vi "禹山叶绿素a校准.vi"() -> ()   [LabVIEW 2016, in "斯坦道多参数.lvlib"]
uses:
  <vilib>/Utility/miscctls.llb/LVPointTypeDef.ctl
  <vilib>/Analysis/NI_AALBase.lvlib
  <vilib>/Analysis/NI_AALPro.lvlib
  <vilib>/Utility/config.llb/NI_LVConfig.lvlib
panel:
  out "通讯状态":string
  out "第二点校准值":dbl
  out "第一点校准值":dbl
  out "最小值":sgl format="%.2g"
  out "最大值":sgl format="%.2g"
  in  "校准停止":bool
  in  "校准模式":enum16{"两点校准", "单点校准"}(ring)
  in  "标液2":dbl
  in  "标液1":dbl
  out "波形图表":sgl(graph) caption="历史曲线"
  out "温度测量值":dbl caption="温度" format="%#.2f"
  out "变异系数":dbl format="%.6g"
  out "standard deviation":dbl caption="标准差" format="%0.2f"
  out "mean":dbl caption="均值" format="%0.2f"
  out "提示":string
  in  "校准启动":bool
  out "测试值":dbl format="%#.2f"
  out "电极斜率":dbl format="%#.6f"
  out "电极零点":dbl format="%#.6f"
  # "叶绿素a电极设定"
  # "请选择校准模式:"
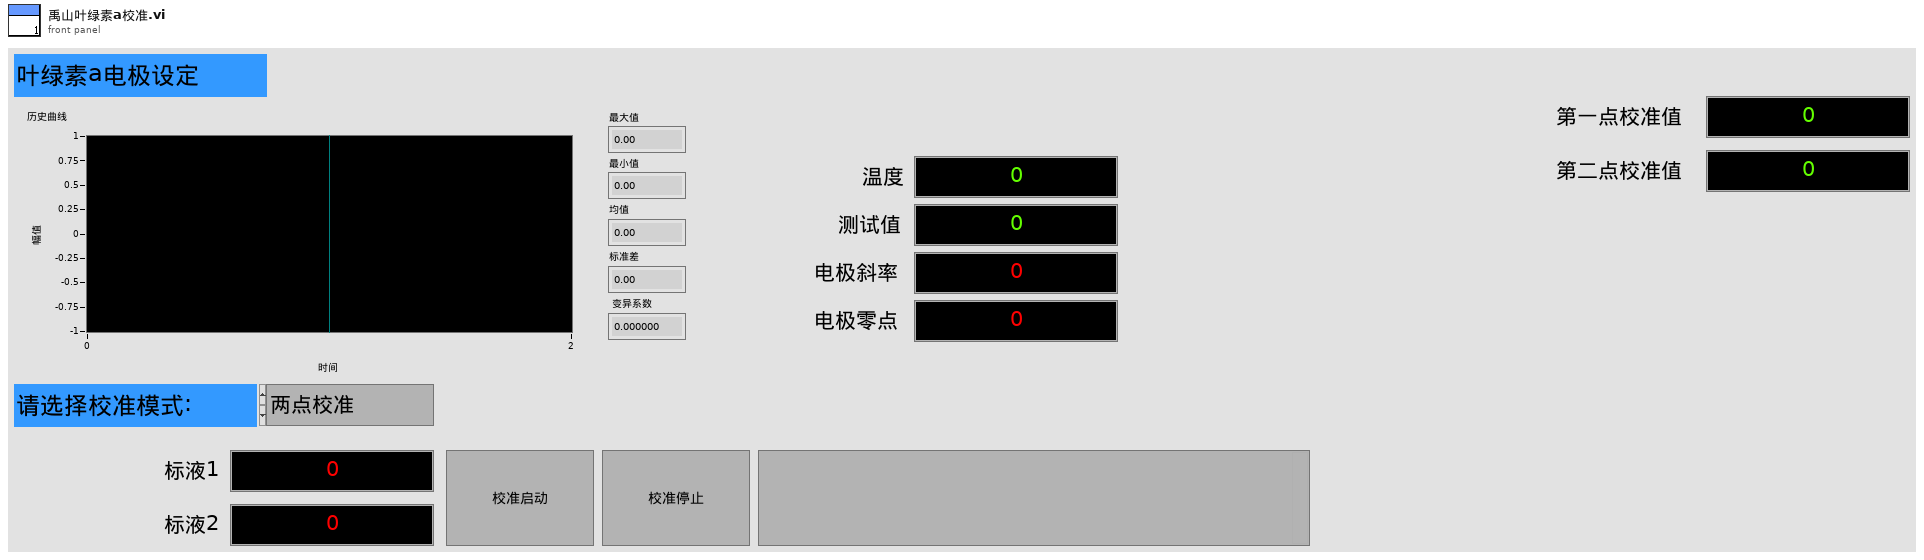
[diagram p1: front panel]
types:
  T1 = typedef "斯坦道多参数.lvlib/校准步骤.ctl" = enum16{"待机", "放置第一点标液", "第一点校准启动", "第一点校准写入", "第一点校准失败", "放置第二点标液", "第二点校准启动", "第二点校准写入", "第二点校准失败", "放置第三点标液", "第三点校准启动", "第三点校准写入", "第三点校准失败", "校准结果写入", "校准结束"}
  T2 = typedef "LVPointTypeDef.ctl" = cluster{"Horizontal":i16, "Vertical":i16}
  T3 = typedef "NI_LVConfig.lvlib/Config Data RefNum.ctl" = refnum<k1>
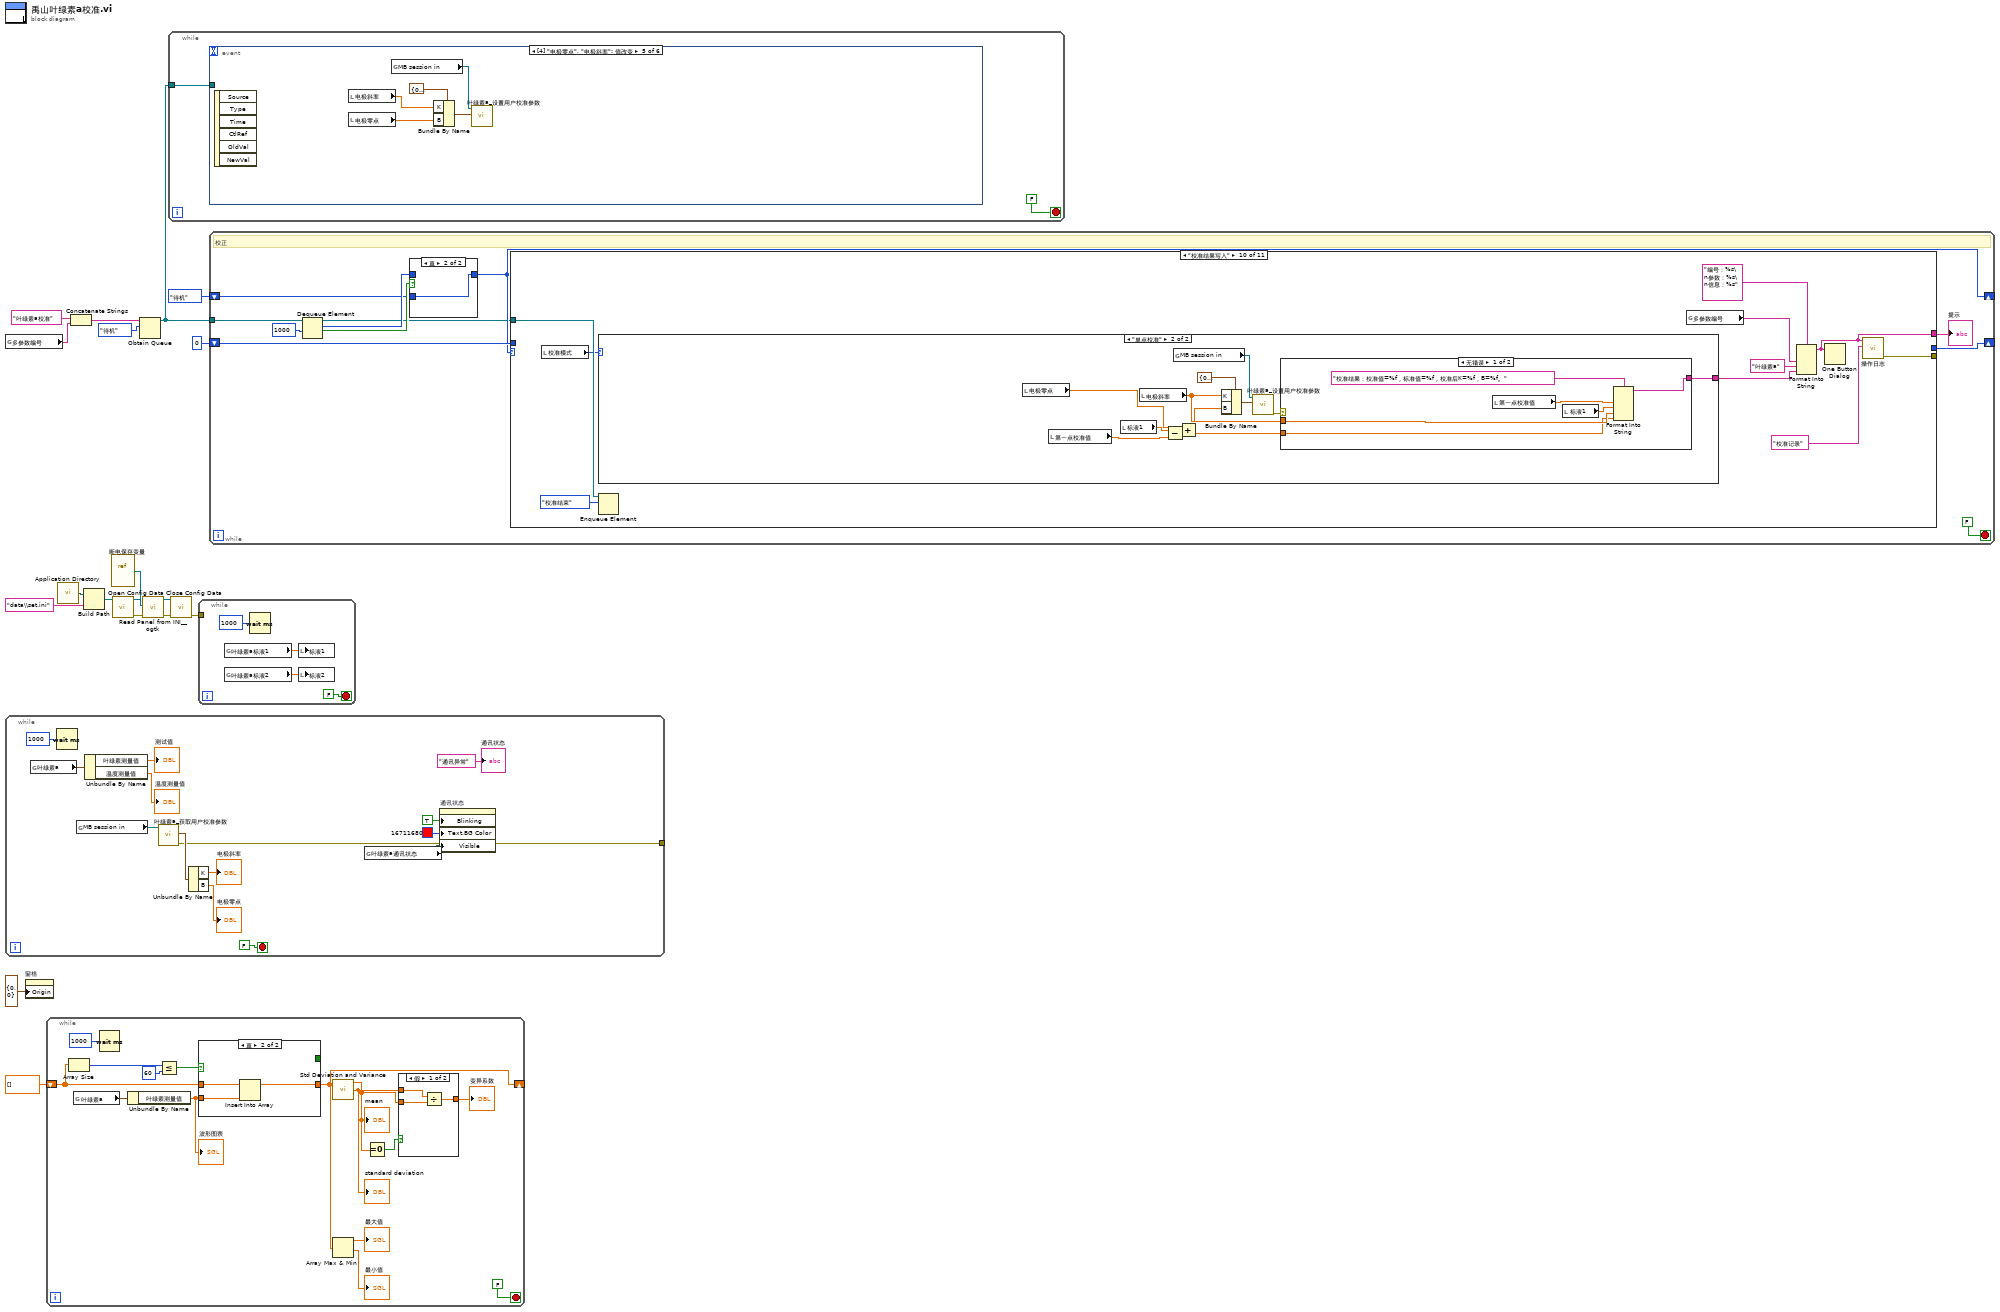
[diagram p0: block diagram]
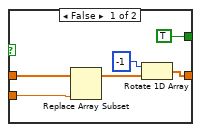
[diagram p3: hidden frame]
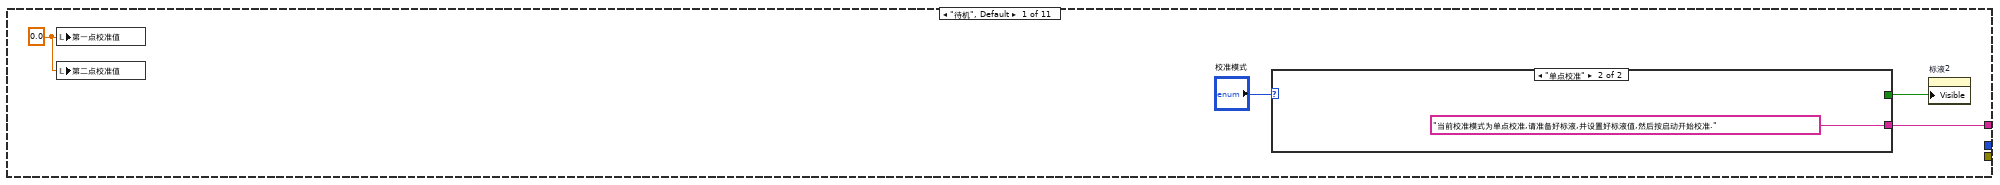
[diagram p5: hidden frame]
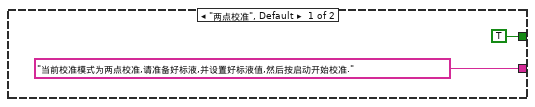
[diagram p6: hidden frame]
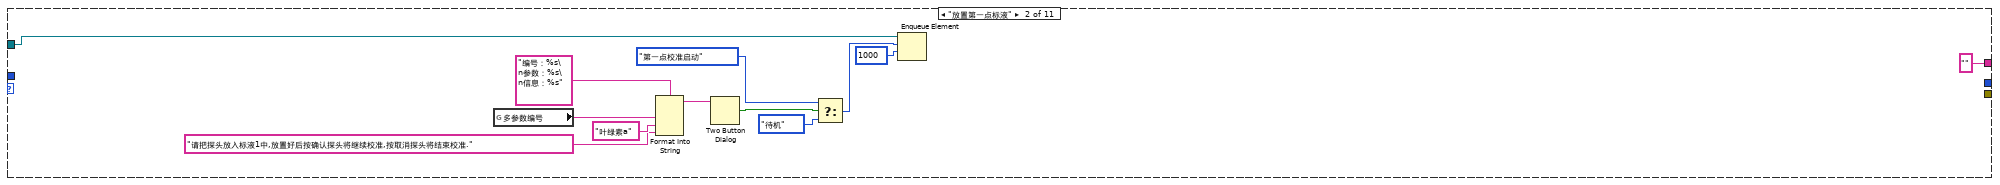
[diagram p7: hidden frame]
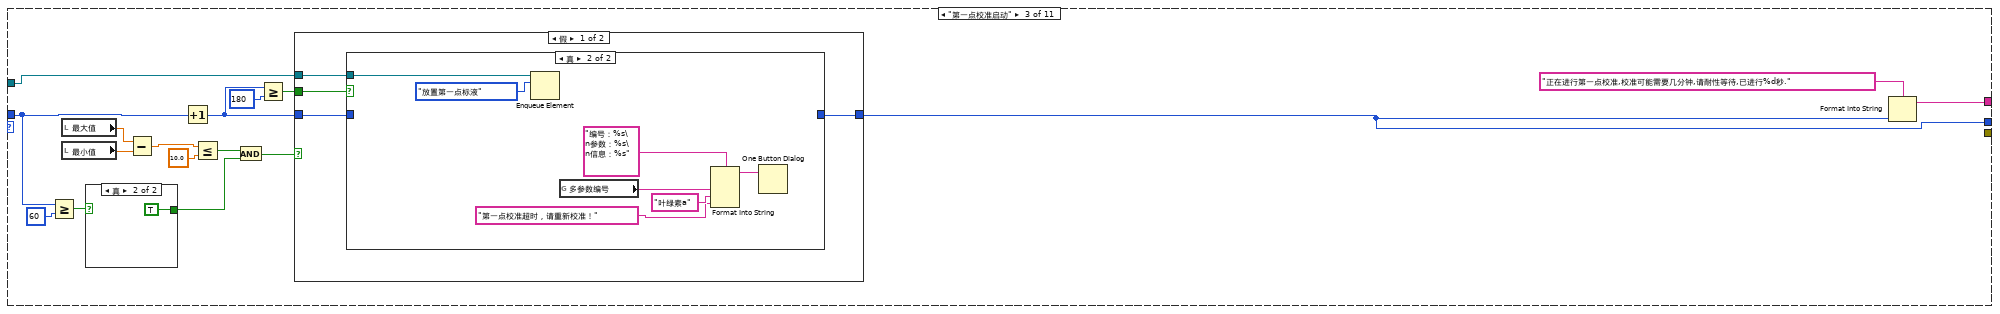
[diagram p8: hidden frame]
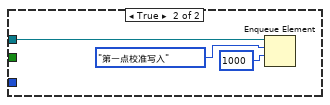
[diagram p10: hidden frame]
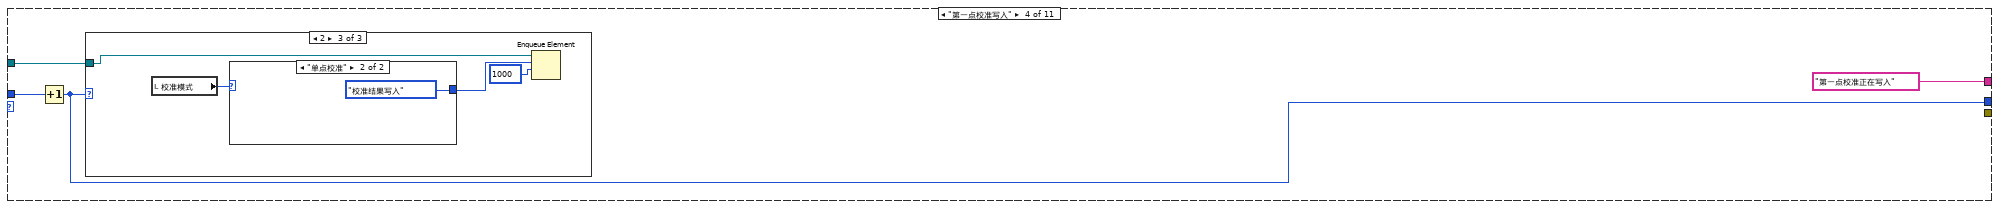
[diagram p12: hidden frame]
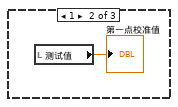
[diagram p14: hidden frame]
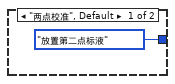
[diagram p15: hidden frame]
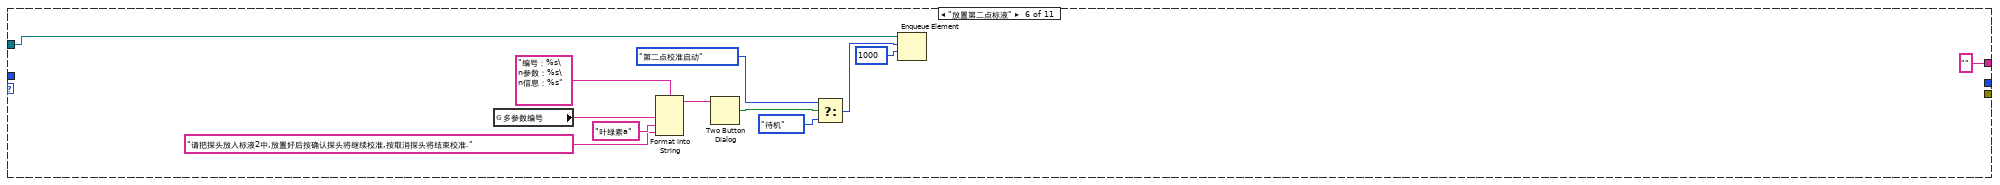
[diagram p17: hidden frame]
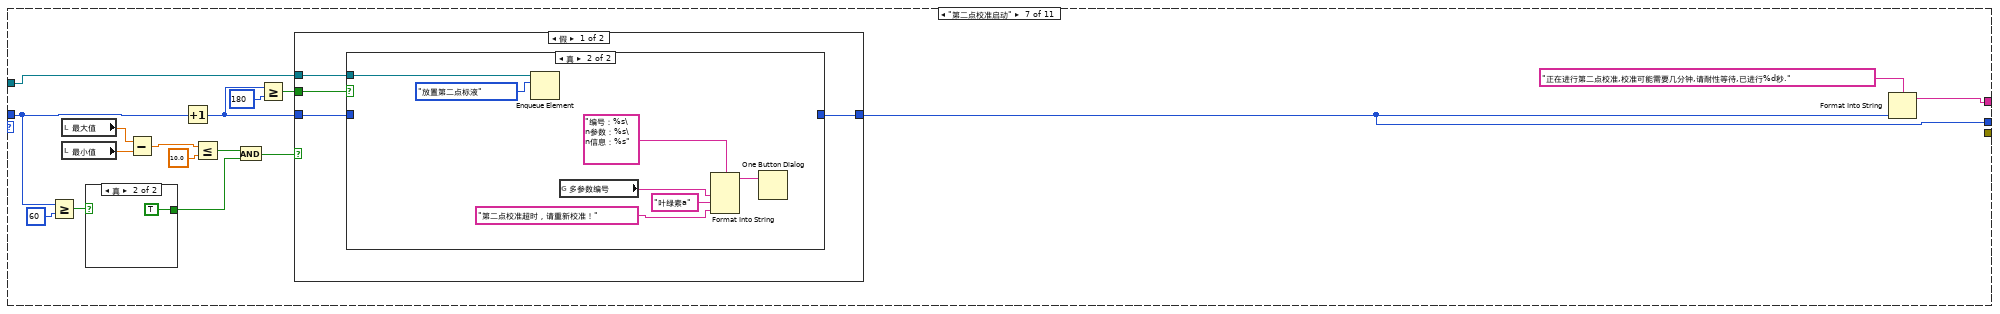
[diagram p18: hidden frame]
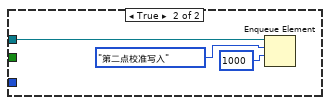
[diagram p20: hidden frame]
diagram:
  n1 = global read "多参数全局变量.vi" "多参数编号"() -> (w1:string)
  n2 = while {
    tunnel: [w27] -> _
    stop <- FALSE stop-if-true
    n3 = global read "禹山过程全局变量.vi" "叶绿素a"() -> (w24:cluster{"温度测量值":sgl, "叶绿素测量值":sgl, "错误标志":u16})
    n4 = Wait (ms)(milliseconds to wait=u32 1000 ("等待时间（毫秒）")) -> ()  [unwired: 1 out]
    n5 = global read "多参数全局变量.vi" "MB session in"() -> (w23:refnum<class "MB_Master.lvclass">)
    n6 = Unbundle By Name(w24) -> ("叶绿素测量值"=→"测试值":sgl, "温度测量值"=→"温度测量值":sgl)
    n7 = call "叶绿素a_获取用户校准参数.vi"("MB session in"=w23) -> ("error out"=w27:errorcluster, "输出值"=w30:cluster{"K":sgl, "B":sgl})  [unwired: 8 in, 1 out]
    n8 = Unbundle By Name(w30) -> ("K"=→"电极斜率":sgl, "B"=→"电极零点":sgl)
    n9 = global read "多参数全局变量.vi" "叶绿素a通讯状态"() -> (w19:bool)
    n10 = property on="通讯状态" class="Str"("Blinking"=TRUE ("闪烁"), "Text.BG Color"=u32 16711680, "Visible"=w19) -> ()  [unwired: 2 in, 2 out]
    "通讯状态" <- "通讯异常" ("当前串口")
  }
  n11 = property on="窗格" class="Pane"("Origin"=T2 {"Horizontal"=0, "Vertical"=0} ("原点")) -> ()  [unwired: 2 in, 2 out]
  n12 = while {
    shift-right: [w35] -> _
    shift-left: sgl[] [] -> [w43]
    stop <- FALSE stop-if-true
    n13 = Array Size(array=w43) -> (size(s)=w45:i32)
    n14 = global read "禹山过程全局变量.vi" "叶绿素a"() -> (w37:cluster{"温度测量值":sgl, "叶绿素测量值":sgl, "错误标志":u16})
    n15 = Wait (ms)(milliseconds to wait=u32 1000 ("等待时间（毫秒）")) -> ()  [unwired: 1 out]
    n16 = Unbundle By Name(w37) -> ("叶绿素测量值"=w36:sgl)
    "波形图表" <- w36
    n17 = Less Or Equal?(x=w45, y=60) -> (x <= y?=w44:bool)
    n18 = case shown="真" w44 {
      tunnel: w43 -> [w56 w59]
      tunnel: w36 -> [w54 w58]
      tunnel: [w52 w57] -> w35
      tunnel: [TRUE _] -> _
      frame False {
        n19 = Replace Array Subset(array=w56, new element=w54) -> (w55:sgl[])  [unwired: 1 in]
        n20 = Rotate 1D Array(1:w55, 2:-1 ("n")) -> (0:w52:sgl[])
      }
      frame True {
        n21 = Insert Into Array(array=w59, new element=w58) -> (w57:sgl[])  [unwired: 1 in]
      }
    }
    n22 = call <vilib>:"Std Deviation and Variance.vi"("X"=w35) -> ("mean"=w38:dbl, "standard deviation"=w39:dbl)  [unwired: 1 in, 1 out]
    "standard deviation" <- w39
    "mean" <- w38
    n23 = Array Max & Min(array=w35) -> (max value=→"最大值":sgl, min value=→"最小值":sgl)  [unwired: 2 out]
    n24 = Equal To 0?(x=w38) -> (x = 0?=w42:bool)
    n25 = case shown="假" w42 {
      tunnel: w39 -> [w50 _]
      tunnel: [w49 _] -> w41
      tunnel: w38 -> [w48 _]
      frame False {
        n26 = Divide(x=w50, y=w48) -> (x/y=w49:dbl)
      }
      frame True {
      }
    }
    "变异系数" <- w41
  }
  n27 = call <vilib>:"Application Directory.vi"() -> ("Application Directory"=w8:path)
  n28 = Concatenate Strings("叶绿素a校准" ("名称（未命名）"), w1) -> (w2:string)
  n29 = Build Path(base path=w8, name or relative path="data\\set.ini" ("名称或相对路径")) -> (appended path=w9:path)
  n30 = vi-ref "断电保存变量.vi"() -> (w11:refnum<vi>)
  n31 = call <vilib>:"Open Config Data.vi"("configuration file path"=w9) -> ("error out"=w5:errorcluster, "refnum"=w4:T3)  [unwired: 8 in, 1 out]
  n32 = Obtain Queue(name (unnamed)=w2, element data type=校准步骤."待机" ("枚举")) -> (queue out=w12:refnum<queue>)  [unwired: 3 in, 2 out]
  n33 = call <userlib>:"Read Panel from INI__ogtk.vi"("error in (no error)"=w5, "VI ref"=w11, "refnum"=w4) -> ("error out"=w7:errorcluster, "refnum out"=w6:T3)  [unwired: 7 in]
  n34 = while {
    tunnel: w12 -> [w60]
    stop <- FALSE stop-if-true
    n35 = event shown="[4] \"电极零点\", \"电极斜率\": 值改变" {
      selector: _ -> [_ _ _ _ _ _]
      dyn-events: _ -> [_ _ _ _ _ _]
      timeout: _ -> [_ _ _ _ _ _]
      tunnel: w60 -> [_ w63 w67 _ _ _]
      event Timeout {
        n36 = event-data() -> ()  [unwired: 1 in, 3 out]
      }
      event "校准启动": Value Change {
        n37 = event-data() -> ()  [unwired: 1 in, 6 out]
        n38 = Enqueue Element(queue=w63, element=校准步骤."放置第一点标液" ("元素")) -> ()  [unwired: 2 in, 3 out]
      }
      event "校准停止": Value Change {
        n39 = event-data() -> ()  [unwired: 1 in, 6 out]
        n40 = Flush Queue(queue=w67) -> (queue out=w64:refnum<queue>)  [unwired: 1 in, 2 out]
        n41 = Enqueue Element(queue=w64, element=校准步骤."待机" ("元素"), timeout in ms (-1)=1000 ("超时毫秒(-1)")) -> ()  [unwired: 1 in, 3 out]
      }
      event "电极零点", "电极斜率", "标液1", "标液2": Mouse Down {
        n42 = event-data() -> ("CtlRef"=w68:refnum<vi>)  [unwired: 1 in, 7 out]
        n43 = property class="DigNum (严格)"(reference=w68) -> (reference out=w69:refnum<vi>, "Value"=w70:dbl)  [unwired: 1 in, 1 out]
        n44 = call "数字键盘.vi"("OldNumber"=w70) -> ("NewNumber"=w71:dbl)  [unwired: 1 in]
        n45 = property class="DigNum (严格)"(reference=w69, "Val(Sgnl)"=w71) -> ()  [unwired: 1 in, 2 out]
      }
      event "电极零点", "电极斜率": Value Change {
        n46 = event-data() -> ()  [unwired: 1 in, 6 out]
        n47 = local read "电极斜率"() -> (w74:dbl)
        n48 = local read "电极零点"() -> (w73:dbl)
        n49 = global read "多参数全局变量.vi" "MB session in"() -> (w72:refnum<class "MB_Master.lvclass">)
        n50 = Bundle By Name(cluster=cluster{"K":sgl, "B":sgl} {"K"=0.0, "B"=0.0} ("用户校准参数"), "K"=w74, "B"=w73) -> (w75:cluster{"K":sgl, "B":sgl})
        n51 = call "叶绿素a_设置用户校准参数.vi"("用户校准参数"=w75, "MB session in"=w72) -> ()  [unwired: 8 in, 2 out]
      }
      event "标液1", "标液2": Value Change {
        n52 = event-data() -> ()  [unwired: 1 in, 6 out]
        n53 = flat-sequence {
          frame #0 {
            n54 = global write "断电保存变量.vi" "叶绿素a标液1"("标液1") -> ()
            n55 = global write "断电保存变量.vi" "叶绿素a标液2"("标液2") -> ()
          }
          frame #1 {
            n56 = call <vilib>:"Application Directory.vi"() -> ("Application Directory"=w88:path)
            n57 = Build Path(base path=w88, name or relative path="data\\set.ini" ("名称或相对路径")) -> (appended path=w87:path)
            n58 = call <vilib>:"Open Config Data.vi"("configuration file path"=w87) -> ("error out"=w91:errorcluster, "refnum"=w92:T3)  [unwired: 8 in, 1 out]
            n59 = vi-ref "断电保存变量.vi"() -> (w85:refnum<vi>)
            n60 = call <userlib>:"Write Panel to INI__ogtk.vi"("error in (no error)"=w91, "VI ref"=w85, "refnum"=w92) -> ("error out"=w89:errorcluster, "refnum out"=w90:T3)  [unwired: 7 in]
            n61 = call <vilib>:"Close Config Data.vi"("error in (no error)"=w89, "refnum"=w90) -> ("error out"=w81:errorcluster, "file path"=w82:path)  [unwired: 8 in]
            n62 = Open/Create/Replace File(file path (use dialog)=w82, error in=w81) -> (refnum out=w83:refnum<file>, error out=w84:errorcluster)  [unwired: 4 in, 1 out]
            n63 = Flush File(refnum=w83, error in=w84) -> (refnum out=w79:refnum<file>, error out=w80:errorcluster)
            n64 = Close File(refnum=w79, error in=w80) -> ()  [unwired: 2 out]
          }
        }
      }
    }
  }
  n65 = call <vilib>:"Close Config Data.vi"("error in (no error)"=w7, "refnum"=w6) -> ("error out"=w3:errorcluster)  [unwired: 8 in, 1 out]
  n66 = while {
    tunnel: w3 -> [_]
    stop <- FALSE stop-if-true
    n67 = global read "断电保存变量.vi" "叶绿素a标液1"() -> (w94:dbl)
    n68 = global read "断电保存变量.vi" "叶绿素a标液2"() -> (w93:dbl)
    n69 = Wait (ms)(milliseconds to wait=u32 1000 ("等待时间（毫秒）")) -> ()  [unwired: 1 out]
    n70 = local write "标液1"(w94) -> ()
    n71 = local write "标液2"(w93) -> ()
  }
  n72 = while "While循环" {
    shift-right: [w98] -> _
    shift-left: 校准步骤."待机" ("枚举") -> [w99]
    shift-right: [w105] -> _
    shift-left: 0 -> [w106]
    tunnel: w12 -> [w103]
    stop <- FALSE stop-if-true
    # "校正"
    n73 = Dequeue Element(queue=w103, timeout in ms (-1)=1000 ("超时毫秒(-1)")) -> (queue out=w97:refnum<queue>, element=w100:T1, timed out?=w101:bool)  [unwired: 1 in, 1 out]
    n74 = case shown="真" w101 {
      tunnel: w100 -> [w108 _]
      tunnel: [w108 w109] -> w98
      tunnel: w99 -> [_ w109]
      frame False {
      }
      frame True {
      }
    }
    n75 = case shown="\"校准结果写入\"" w98 {
      tunnel: [w113 "" ("提示") w144 "第一点校准正在写入" ("提示") _ "" ("提示") w200 "第二点校准正在写入" ("提示") _ w227 w283] -> w104
      tunnel: w106 -> [_ _ w138 w164 _ _ w194 w220 _ _ _]
      tunnel: [_ _ w129 w163 _ _ w185 w219 _ _ _] -> w105
      tunnel: w97 -> [_ w128 w132 w162 _ w184 w188 w218 _ w235 _]
      tunnel: [_ _ _ _ _ _ _ _ _ w232 _] -> _
      frame "待机", Default {
        w110 = 0.0 ("第一点校准值")
        n76 = local write "第一点校准值"(w110) -> ()
        n77 = local write "第二点校准值"(w110) -> ()
        n78 = case shown="\"单点校准\"" "校准模式" {
          tunnel: ["当前校准模式为两点校准,请准备好标液,并设置好标液值,然后按启动开始校准." ("提示") "当前校准模式为单点校准,请准备好标液,并设置好标液值,然后按启动开始校准." ("提示")] -> w113
          tunnel: [TRUE ("可见") _] -> w111
          frame "两点校准", Default {
          }
          frame "单点校准" {
          }
        }
        n79 = property on="标液2" class="DigNum (严格)"("Visible"=w111) -> ()  [unwired: 2 in, 2 out]
      }
      frame "放置第一点标液" {
        n80 = global read "多参数全局变量.vi" "多参数编号"() -> (w120:string)
        n81 = Format Into String(format string="编号：%s\n参数：%s\n信息：%s" ("格式字符串"), w120, "叶绿素a" ("输入 2"), "请把探头放入标液1中,放置好后按确认探头将继续校准,按取消探头将结束校准." ("消息")) -> (resulting string=w117:string)  [unwired: 2 in, 1 out]
        n82 = Two Button Dialog(message=w117) -> (T button?=w126:bool)  [unwired: 2 in]
        n83 = Select(t=校准步骤."第一点校准启动" ("元素"), s=w126, f=校准步骤."待机" ("元素")) -> (s? t:f=w123:T1)
        n84 = Enqueue Element(queue=w128, element=w123, timeout in ms (-1)=1000 ("超时毫秒(-1)")) -> ()  [unwired: 1 in, 3 out]
      }
      frame "第一点校准启动" {
        n85 = Greater Or Equal?(x=w138, y=60) -> (x >= y?=w139:bool)
        n86 = local read "最大值"() -> (w135:sgl)
        n87 = local read "最小值"() -> (w136:sgl)
        n88 = case shown="真" w139 {
          tunnel: [_ TRUE] -> w137
          frame False {
          }
          frame True {
          }
        }
        n89 = Subtract(x=w135, y=w136) -> (x-y=w134:sgl)
        n90 = Increment(x=w138) -> (x+1=w130:i32)
        n91 = Less Or Equal?(x=w134, y=10.0) -> (x <= y?=w142:bool)
        n92 = And(x=w142, y=w137) -> (x .and. y?=w133:bool)
        n93 = Greater Or Equal?(x=w130, y=180) -> (x >= y?=w131:bool)
        n94 = case shown="假" w133 {
          tunnel: w132 -> [w148 w160]
          tunnel: w131 -> [w149 _]
          tunnel: w130 -> [w147 _]
          tunnel: [w146 _] -> w129
          frame False {
            n95 = case shown="真" w149 {
              tunnel: w148 -> [_ w157]
              tunnel: w147 -> [w150 _]
              tunnel: [w150 _] -> w146
              frame False {
              }
              frame True {
                n96 = Enqueue Element(queue=w157, element=校准步骤."放置第一点标液" ("元素")) -> ()  [unwired: 2 in, 3 out]
                n97 = global read "多参数全局变量.vi" "多参数编号"() -> (w154:string)
                n98 = Format Into String(format string="编号：%s\n参数：%s\n信息：%s" ("格式字符串"), w154, "叶绿素a" ("输入 2"), "第一点校准超时，请重新校准！" ("error source (\" \")")) -> (resulting string=w152:string)  [unwired: 2 in, 1 out]
                n99 = One Button Dialog(message=w152) -> ()  [unwired: 1 in, 1 out]
              }
            }
          }
          frame True {
            n100 = Enqueue Element(queue=w160, element=校准步骤."第一点校准写入" ("元素"), timeout in ms (-1)=1000 ("超时毫秒(-1)")) -> ()  [unwired: 1 in, 3 out]
          }
        }
        n101 = Format Into String(format string="正在进行第一点校准,校准可能需要几分钟,请耐性等待,已进行%d秒." ("格式字符串"), w129) -> (resulting string=w144:string)  [unwired: 2 in, 1 out]
      }
      frame "第一点校准写入" {
        n102 = Increment(x=w164) -> (x+1=w163:i32)
        n103 = case shown="2" w163 {
          tunnel: w162 -> [_ _ w170]
          frame 0, Default {
          }
          frame 1 {
            n104 = local read "测试值"() -> (→"第一点校准值":dbl)
          }
          frame 2 {
            n105 = local read "校准模式"() -> (w169:enum16{"两点校准", "单点校准"})
            n106 = case shown="\"单点校准\"" w169 {
              tunnel: [校准步骤."放置第二点标液" ("元素") 校准步骤."校准结果写入" ("元素")] -> w168
              frame "两点校准", Default {
              }
              frame "单点校准" {
              }
            }
            n107 = Enqueue Element(queue=w170, element=w168, timeout in ms (-1)=1000 ("超时毫秒(-1)")) -> ()  [unwired: 1 in, 3 out]
          }
        }
      }
      frame "第一点校准失败" {
      }
      frame "放置第二点标液" {
        n108 = global read "多参数全局变量.vi" "多参数编号"() -> (w176:string)
        n109 = Format Into String(format string="编号：%s\n参数：%s\n信息：%s" ("格式字符串"), w176, "叶绿素a" ("输入 2"), "请把探头放入标液2中,放置好后按确认探头将继续校准,按取消探头将结束校准." ("消息")) -> (resulting string=w173:string)  [unwired: 2 in, 1 out]
        n110 = Two Button Dialog(message=w173) -> (T button?=w182:bool)  [unwired: 2 in]
        n111 = Select(t=校准步骤."第二点校准启动" ("元素"), s=w182, f=校准步骤."待机" ("元素")) -> (s? t:f=w179:T1)
        n112 = Enqueue Element(queue=w184, element=w179, timeout in ms (-1)=1000 ("超时毫秒(-1)")) -> ()  [unwired: 1 in, 3 out]
      }
      frame "第二点校准启动" {
        n113 = Greater Or Equal?(x=w194, y=60) -> (x >= y?=w195:bool)
        n114 = local read "最大值"() -> (w191:sgl)
        n115 = local read "最小值"() -> (w192:sgl)
        n116 = case shown="真" w195 {
          tunnel: [_ TRUE] -> w193
          frame False {
          }
          frame True {
          }
        }
        n117 = Subtract(x=w191, y=w192) -> (x-y=w190:sgl)
        n118 = Increment(x=w194) -> (x+1=w186:i32)
        n119 = Less Or Equal?(x=w190, y=10.0) -> (x <= y?=w198:bool)
        n120 = And(x=w198, y=w193) -> (x .and. y?=w189:bool)
        n121 = Greater Or Equal?(x=w186, y=180) -> (x >= y?=w187:bool)
        n122 = case shown="假" w189 {
          tunnel: w188 -> [w204 w216]
          tunnel: w187 -> [w205 _]
          tunnel: w186 -> [w203 _]
          tunnel: [w202 _] -> w185
          frame False {
            n123 = case shown="真" w205 {
              tunnel: w204 -> [_ w213]
              tunnel: w203 -> [w206 _]
              tunnel: [w206 _] -> w202
              frame False {
              }
              frame True {
                n124 = Enqueue Element(queue=w213, element=校准步骤."放置第二点标液" ("元素")) -> ()  [unwired: 2 in, 3 out]
                n125 = global read "多参数全局变量.vi" "多参数编号"() -> (w210:string)
                n126 = Format Into String(format string="编号：%s\n参数：%s\n信息：%s" ("格式字符串"), w210, "叶绿素a" ("输入 2"), "第二点校准超时，请重新校准！" ("error source (\" \")")) -> (resulting string=w208:string)  [unwired: 2 in, 1 out]
                n127 = One Button Dialog(message=w208) -> ()  [unwired: 1 in, 1 out]
              }
            }
          }
          frame True {
            n128 = Enqueue Element(queue=w216, element=校准步骤."第二点校准写入" ("元素"), timeout in ms (-1)=1000 ("超时毫秒(-1)")) -> ()  [unwired: 1 in, 3 out]
          }
        }
        n129 = Format Into String(format string="正在进行第二点校准,校准可能需要几分钟,请耐性等待,已进行%d秒." ("格式字符串"), w185) -> (resulting string=w200:string)  [unwired: 2 in, 1 out]
      }
      frame "第二点校准写入" {
        n130 = Increment(x=w220) -> (x+1=w219:i32)
        n131 = case shown="2" w219 {
          tunnel: w218 -> [_ _ w225]
          frame 0, Default {
          }
          frame 1 {
            n132 = local read "测试值"() -> (→"第二点校准值":dbl)
          }
          frame 2 {
            n133 = Enqueue Element(queue=w225, element=校准步骤."校准结果写入" ("元素"), timeout in ms (-1)=1000 ("超时毫秒(-1)")) -> ()  [unwired: 1 in, 3 out]
          }
        }
      }
      frame "第二点校准失败" {
      }
      frame "校准结果写入" {
        n134 = local read "校准模式"() -> (w233:enum16{"两点校准", "单点校准"})
        n135 = case shown="\"单点校准\"" w233 {
          tunnel: [w243 w271] -> w228
          frame "两点校准", Default {
            n136 = local read "第一点校准值"() -> (w254:dbl)
            n137 = local read "第二点校准值"() -> (w253:dbl)
            n138 = local read "标液1"() -> (w251:dbl)
            n139 = local read "标液2"() -> (w250:dbl)
            n140 = Insert Into Array(array=dbl[] [] ("Weight"), new element #1=w251, new element #2=w250) -> (w249:dbl[])  [unwired: 1 in]
            n141 = Insert Into Array(array=dbl[] [] ("Weight"), new element #1=w254, new element #2=w253) -> (w248:dbl[])  [unwired: 1 in]
            n142 = local read "电极零点"() -> (w240:dbl)
            n143 = call <vilib>:"Linear Fit.vi"("Y"=w249, "X"=w248) -> ("slope"=w239:dbl, "intercept"=w237:dbl)  [unwired: 9 in, 3 out]
            n144 = local read "电极斜率"() -> (w241:dbl)
            n145 = Multiply(x=w239, y=w240) -> (x*y=w238:dbl)
            n146 = Multiply(x=w241, y=w239) -> (x*y=w242:dbl)
            n147 = Add(x=w237, y=w238) -> (x+y=w236:dbl)
            n148 = global read "多参数全局变量.vi" "MB session in"() -> (w247:refnum<class "MB_Master.lvclass">)
            n149 = Bundle By Name(cluster=cluster{"K":sgl, "B":sgl} {"K"=0.0, "B"=0.0} ("用户校准参数"), "K"=w242, "B"=w236) -> (w246:cluster{"K":sgl, "B":sgl})
            n150 = call "叶绿素a_设置用户校准参数.vi"("用户校准参数"=w246, "MB session in"=w247) -> ("error out"=w244:errorcluster)  [unwired: 8 in, 1 out]
            n151 = case shown="无错误" w244 {
              tunnel: w242 -> [w261 _]
              tunnel: w236 -> [w260 _]
              tunnel: [w259 "校准失败"] -> w243
              frame No Error {
                n152 = local read "第一点校准值"() -> (w262:dbl)
                n153 = local read "第二点校准值"() -> (w263:dbl)
                n154 = local read "标液1"() -> (w257:dbl)
                n155 = local read "标液2"() -> (w256:dbl)
                n156 = Format Into String(format string="校准结果：第一点校准值=%f，第一点标准值=%f；第二点校准值=%f，第二点标准值=%f；校准后K=%f；B=%f。" ("提示"), w262, w257, w263, w256, w261, w260) -> (resulting string=w259:string)  [unwired: 2 in, 1 out]
              }
              frame Error {
              }
            }
          }
          frame "单点校准" {
            n157 = local read "电极零点"() -> (w265:dbl)
            n158 = local read "第一点校准值"() -> (w269:dbl)
            n159 = local read "标液1"() -> (w268:dbl)
            n160 = local read "电极斜率"() -> (w270:dbl)
            n161 = Subtract(x=w268, y=w269) -> (x-y=w267:dbl)
            n162 = global read "多参数全局变量.vi" "MB session in"() -> (w275:refnum<class "MB_Master.lvclass">)
            n163 = Add(x=w265, y=w267) -> (x+y=w266:dbl)
            n164 = Bundle By Name(cluster=cluster{"K":sgl, "B":sgl} {"K"=0.0, "B"=0.0} ("用户校准参数"), "K"=w270, "B"=w266) -> (w274:cluster{"K":sgl, "B":sgl})
            n165 = call "叶绿素a_设置用户校准参数.vi"("用户校准参数"=w274, "MB session in"=w275) -> ("error out"=w272:errorcluster)  [unwired: 8 in, 1 out]
            n166 = case shown="无错误" w272 {
              tunnel: w270 -> [w280 _]
              tunnel: w266 -> [w279 _]
              tunnel: [w278 "校准失败"] -> w271
              frame No Error {
                n167 = local read "第一点校准值"() -> (w281:dbl)
                n168 = local read "标液1"() -> (w276:dbl)
                n169 = Format Into String(format string="校准结果：校准值=%f，标准值=%f，校准后K=%f，B=%f。" ("提示"), w281, w276, w280, w279) -> (resulting string=w278:string)  [unwired: 2 in, 1 out]
              }
              frame Error {
              }
            }
          }
        }
        n170 = Enqueue Element(queue=w235, element=校准步骤."校准结束" ("元素")) -> ()  [unwired: 2 in, 3 out]
        n171 = global read "多参数全局变量.vi" "多参数编号"() -> (w230:string)
        n172 = Format Into String(format string="编号：%s\n参数：%s\n信息：%s" ("格式字符串"), w230, "叶绿素a" ("输入 2"), w228) -> (resulting string=w227:string)  [unwired: 2 in, 1 out]
        n173 = One Button Dialog(message=w227) -> ()  [unwired: 1 in, 1 out]
        n174 = call "操作日志.vi"("table"="校准记录", "日志信息"=w227) -> ("error out"=w232:errorcluster)  [unwired: 9 in]
      }
      frame "校准结束" {
        n175 = local read "提示"() -> (w283:string)
      }
    }
    "提示" <- w104
  }
